vi "Overview.vi"() -> ()   [LabVIEW 2024]
uses:
  Overview_States.ctl
  State Data.ctl
  <vilib>/Plug-In SDKs/Clients/Metadata/Operator.ctl
  <vilib>/Plug-In SDKs/Clients/Metadata/Extension Value.ctl
  <vilib>/Plug-In SDKs/Clients/Metadata/Test Station.ctl
  <vilib>/Plug-In SDKs/Clients/Metadata/Software Item.ctl
  <vilib>/Plug-In SDKs/Clients/Data Store V1/Data Store Client.lvlibp/API/Data Store V1/Test Result.ctl
  <vilib>/Plug-In SDKs/Clients/Metadata/Outcome.ctl
  <vilib>/Plug-In SDKs/Clients/Metadata/Error Information.ctl
  <vilib>/Plug-In SDKs/Clients/Metadata/Step.ctl
  <vilib>/Plug-In SDKs/Clients/Metadata Store V1/Metadata Store Client.lvlibp/API/Metadata Store V1/Register Schema (Path).vi
  <vilib>/Plug-In SDKs/Clients/Metadata Store V1/Metadata Store Client.lvlibp/API/Metadata Store V1/Create Operator.vi
  <vilib>/Plug-In SDKs/Clients/Metadata Store V1/Metadata Store Client.lvlibp/API/Metadata Store V1/Create Alias (Metadata - Operator).vi
  <vilib>/Plug-In SDKs/Clients/Metadata Store V1/Metadata Store Client.lvlibp/API/Metadata Store V1/Create Test Station.vi
  <vilib>/Plug-In SDKs/Clients/Metadata Store V1/Metadata Store Client.lvlibp/API/Metadata Store V1/Create Software Item.vi
  <vilib>/Plug-In SDKs/Clients/Metadata Store V1/Metadata Store Client.lvlibp/API/Metadata Store V1/Query Test Stations.vi
  <vilib>/Plug-In SDKs/Clients/Data Store V1/Data Store Client.lvlibp/API/Data Store V1/Publish Measurement (DBL Analog Waveform).vi
  <vilib>/Plug-In SDKs/Clients/Metadata Store V1/Metadata Store Client.lvlibp/API/Metadata Store V1/Get Operator.vi
  <vilib>/Plug-In SDKs/Clients/Data Store V1/Data Store Client.lvlibp/API/Data Store V1/Read Data from Measurement (DBL Analog Waveform).vi
  <vilib>/Plug-In SDKs/Clients/Metadata Store V1/Metadata Store Client.lvlibp
  <vilib>/Plug-In SDKs/Clients/Data Store V1/Data Store Client.lvlibp
  <vilib>/Plug-In SDKs/Clients/Metadata/NI Metadata Types.lvlib
  <vilib>/measure/NI_MABase.lvlib
panel:
  out "queried data":waveform(dbl)(graph)
  out "log":string
  out "error out":errorcluster
  # "Overview\n\nThis example publishes a waveform along with metadata and extension attributes.\nThen it queries for the published data and displays it."
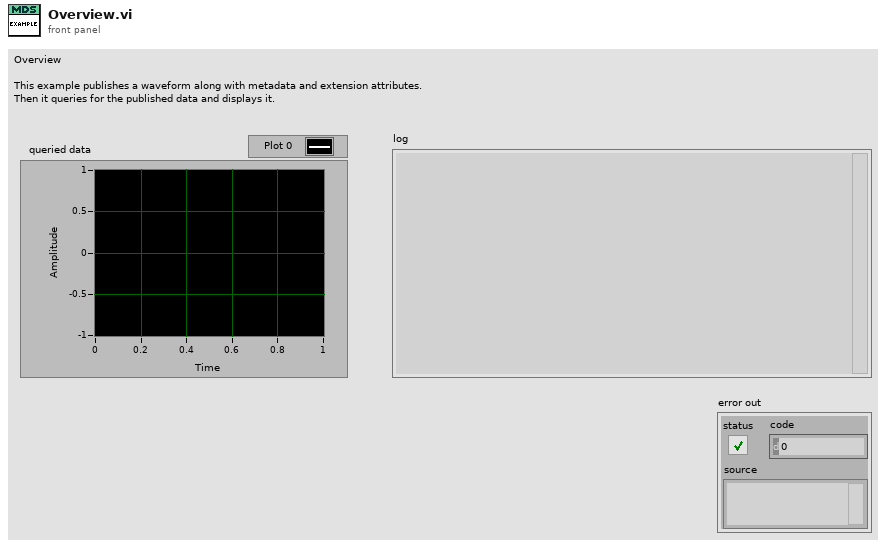
[diagram p1: front panel]
types:
  T1 = typedef "State Data.ctl" = cluster{"schema id":string, "software item ids":string[], "test result id":string, "published measurement id":string}
  T2 = typedef "Overview_States.ctl" = enum16{"Register Metadata Schema", "Create Metadata", "Create Test Result", "Publish Data", "Query Published Data"}
  T3 = enum16{"Register Metadata Schema", "Create Metadata", "Create Test Result", "Publish Data", "Query Published Data"}
  T4 = typedef "NI Metadata Types.lvlib/Extension Value.ctl" = cluster{"name":string, "value":string}
  T5 = typedef "NI Metadata Types.lvlib/Software Item.ctl" = cluster{"product":string, "version":string, "id":string, "link":string, "extension":T4[], "schema id":string}
  T6 = typedef "NI Metadata Types.lvlib/Test Station.ctl" = cluster{"name":string, "asset identifier":string, "id":string, "link":string, "extension":T4[], "schema id":string}
  T7 = typedef "NI Metadata Types.lvlib/Operator.ctl" = cluster{"name":string, "role":string, "id":string, "link":string, "extension":T4[], "schema id":string}
  T8 = typedef "Data Store Client.lvlibp/Test Result.ctl" = cluster{"name":string, "start date time":timestamp, "end date time":timestamp, "outcome":T9, "error information":T10, "id":string, "uut instance id":string, "operator id":string, "test station id":string, "test description id":string, "software item ids":string[], "hardware item ids":string[], "test adapter ids":string[], "link":string, "extension":T4[], "schema id":string}
  T9 = typedef "NI Metadata Types.lvlib/Outcome.ctl" = enum32{"Unspecified", "Passed", "Failed", "Indeterminate"}
  T10 = typedef "NI Metadata Types.lvlib/Error Information.ctl" = cluster{"error code":i32, "message":string, "source":string}
  T11 = typedef "NI Metadata Types.lvlib/Step.ctl" = cluster{"name":string, "step type":string, "start date time":timestamp, "end date time":timestamp, "notes":string, "outcome":T9, "error information":T10, "id":string, "parent step id":string, "test result id":string, "test id":string, "link":string, "extension":T4[], "schema id":string}
  T12 = typedef "Data Store Client.lvlibp/Published Measurement.ctl" = cluster{"parametric index":i32, "name":string, "value type":string, "notes":string, "start date time":timestamp, "end date time":timestamp, "outcome":T9, "error information":T10, "published conditions":T13[], "data moniker":T14, "id":string, "test result id":string, "step id":string, "software item ids":string[], "hardware item ids":string[], "test adapter ids":string[]}
  T13 = typedef "Data Store Client.lvlibp/Published Condition.ctl" = cluster{"name":string, "condition type":string, "moniker":T14, "id":string, "step id":string, "test result id":string}
  T14 = typedef "Data Store Client.lvlibp/Data Moniker.ctl" = cluster{"service location":string, "data source":string, "data instance":i64}
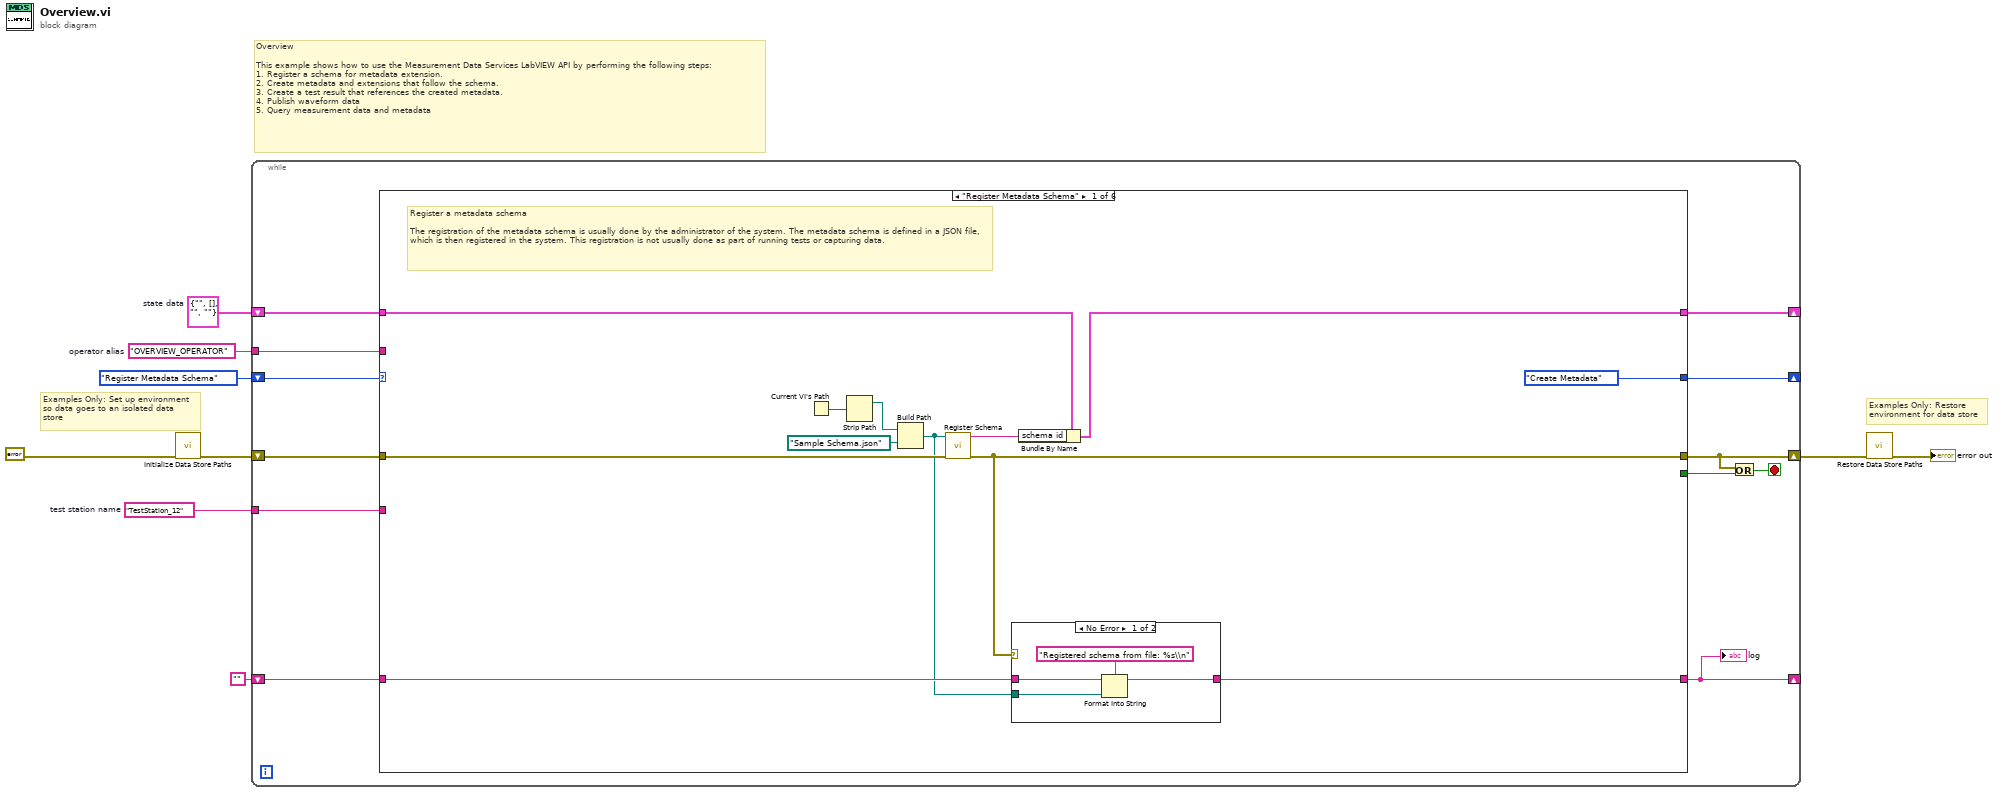
[diagram p0: block diagram]
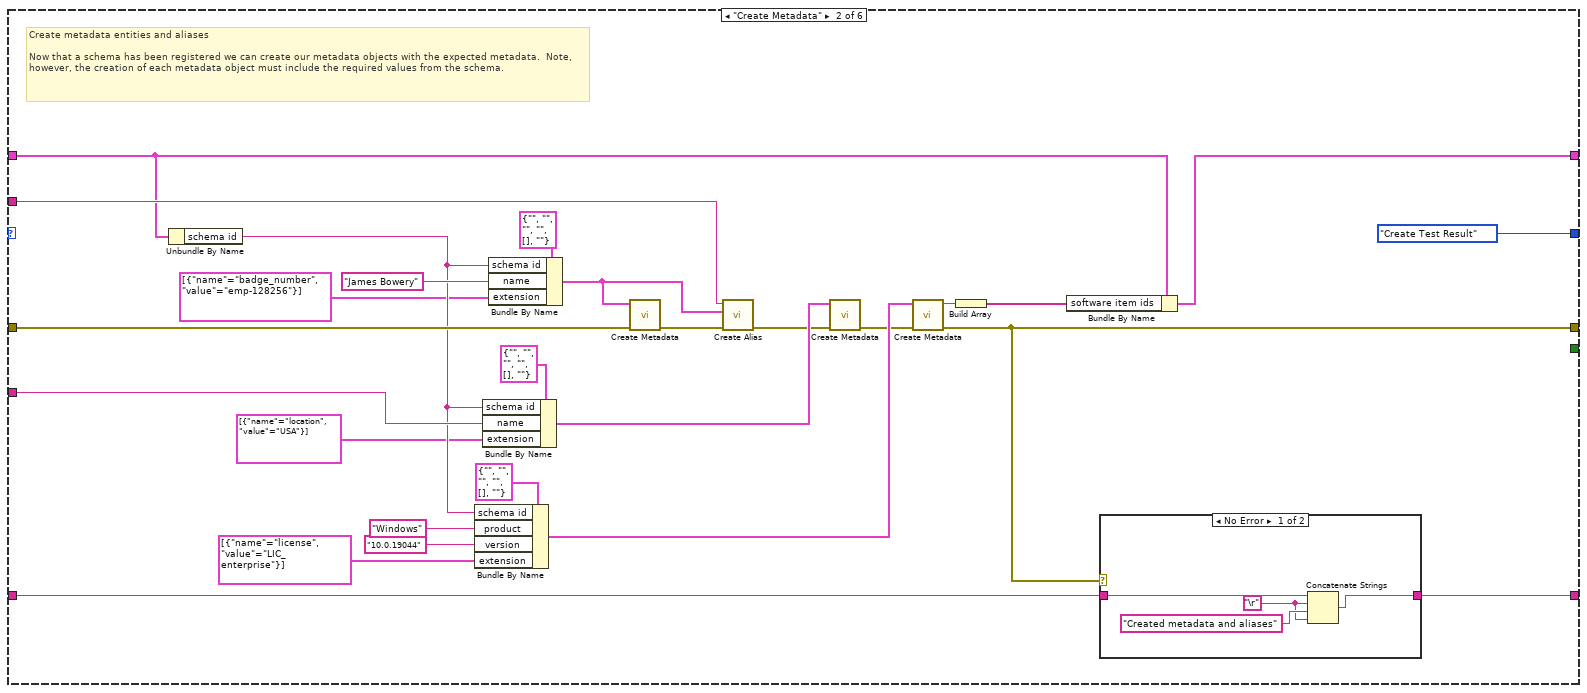
[diagram p3: hidden frame]
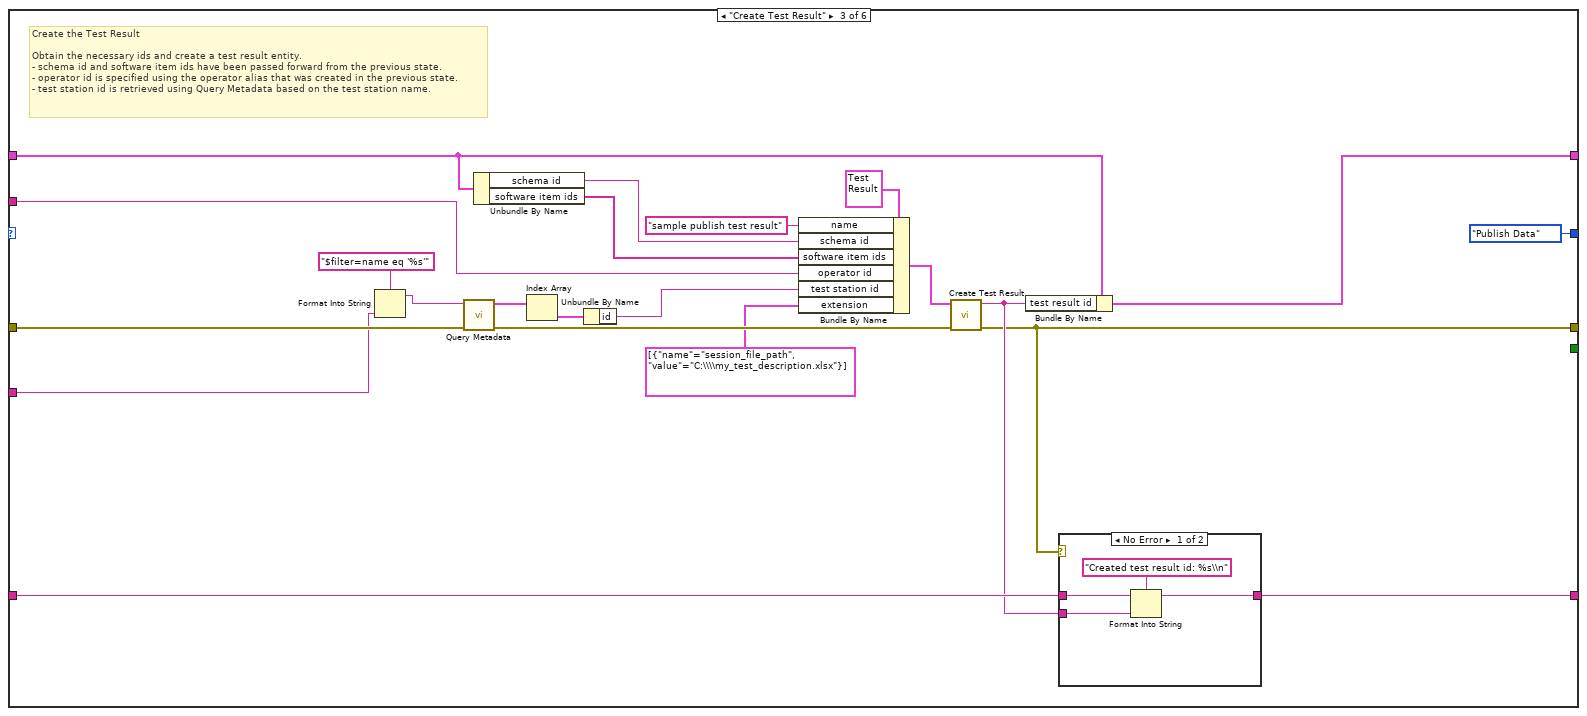
[diagram p5: hidden frame]
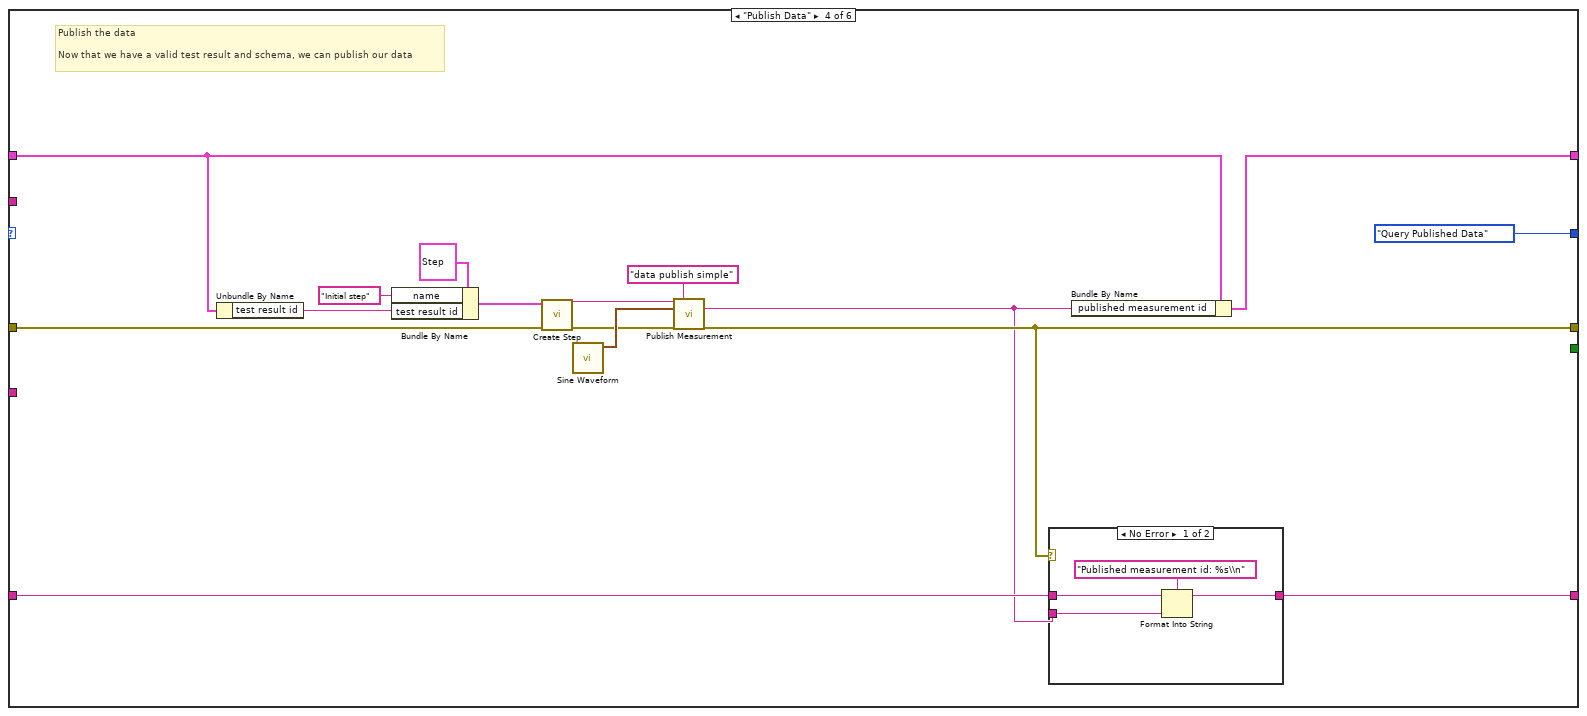
[diagram p7: hidden frame]
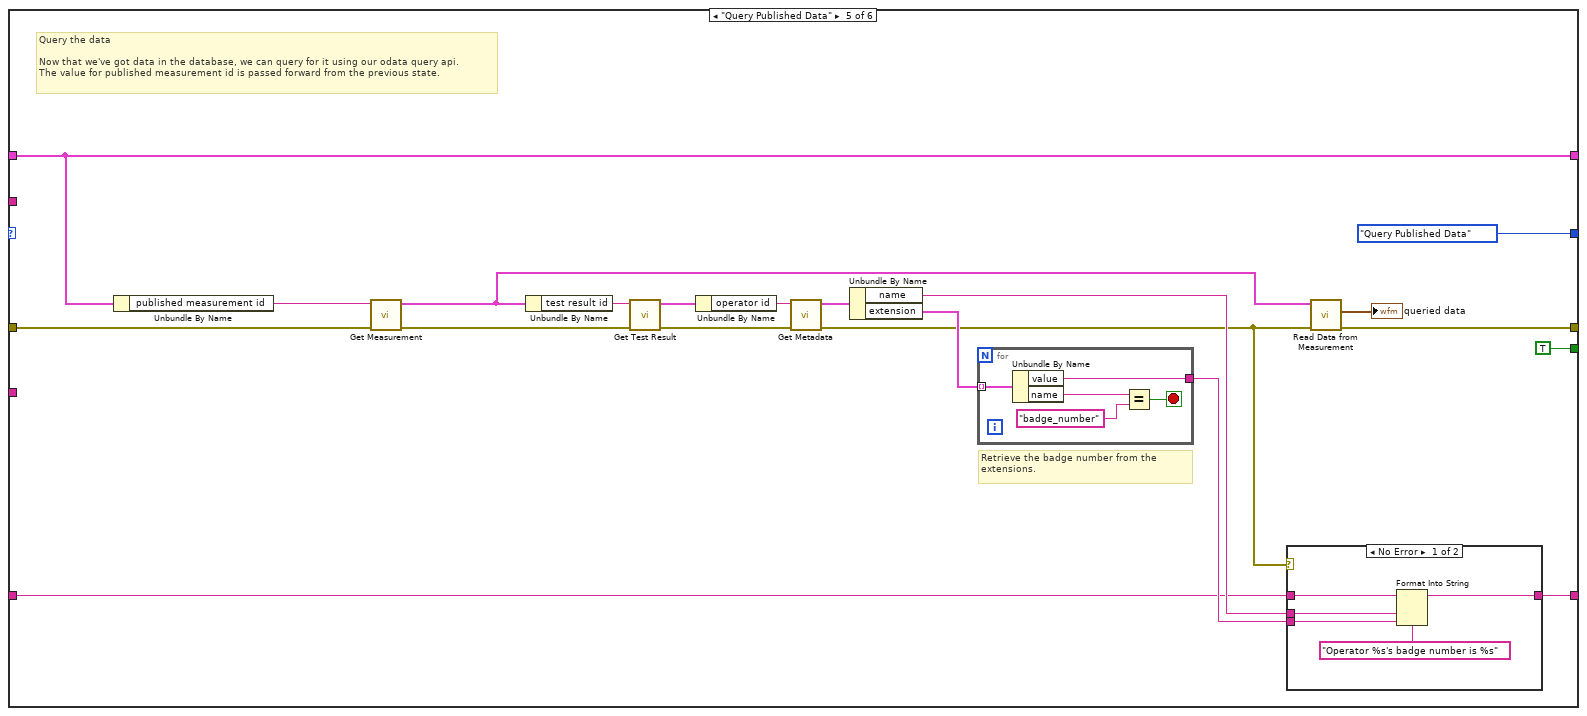
[diagram p9: hidden frame]
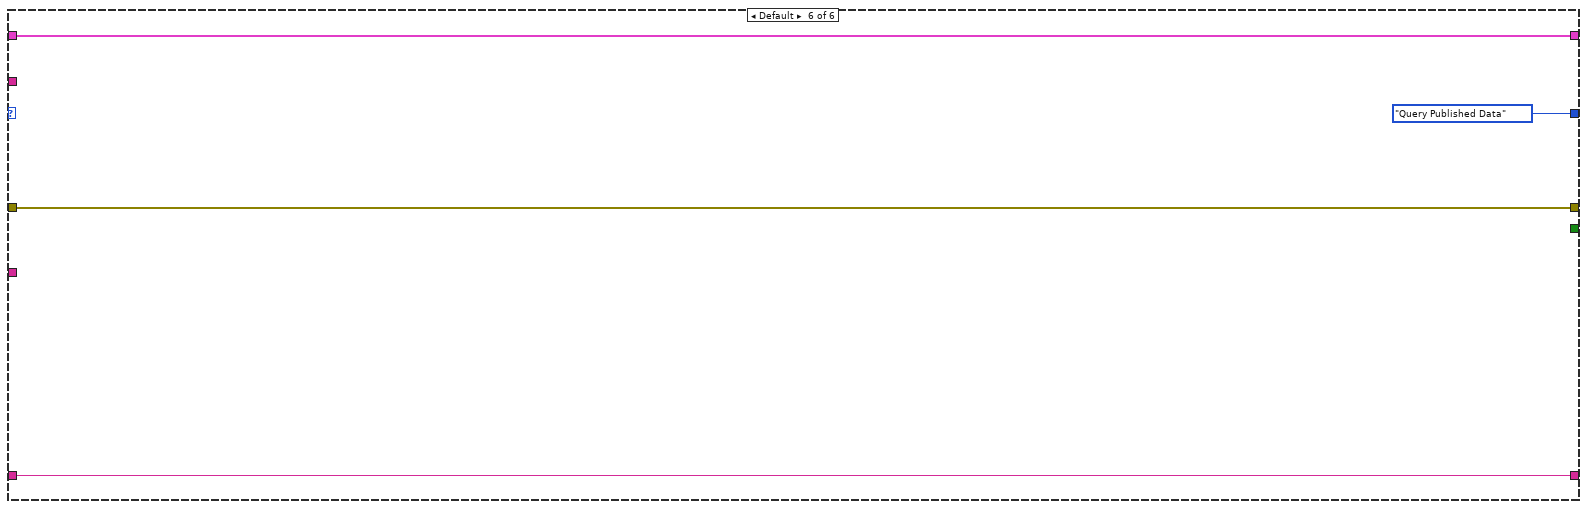
[diagram p11: hidden frame]
diagram:
  w5 = "OVERVIEW_OPERATOR"  # operator alias
  w6 = "TestStation_12"  # test station name
  w7 = T1 {"schema id"="", "software item ids"=[], "test result id"="", "published measurement id"=""}  # state data
  # "Examples Only: Restore\nenvironment for data store"
  # "Examples Only: Set up environment\nso data goes to an isolated data\nstore"
  # "Overview\n\nThis example shows how to use the Measurement Data Services LabVIEW API by performing the following steps:\n1. Register a schema for metadata extension.\n2. Create metadata and extensions that follow the schema.\n3. Create a test result that references the created metadata.\n4. Publish waveform data\n5. Query measurement data and metadata"
  n1 = call "Initialize Data Store Paths.vi"("error in"=errorcluster {"status"=FALSE, "code"=0, "source"=""} ("error out")) -> ("error out"=w3:errorcluster)  [unwired: 10 in]
  n2 = while {
    shift-right: [w18] -> _
    shift-left: Overview_States."Register Metadata Schema" ("state variable") -> [w21]
    shift-right: [w16] -> w2
    shift-left: w3 -> [w20]
    shift-right: [w17] -> _
    shift-left: "" ("log") -> [w19]
    shift-right: [w10] -> _
    shift-left: w7 -> [w13]
    tunnel: w6 -> [w12]
    tunnel: w5 -> [w11]
    stop <- w14 stop-if-true
    n3 = case shown="\"Register Metadata Schema\"" w21 {
      tunnel: [w27 w44 w75 w103 w138 w153] -> w16
      tunnel: w20 -> [w28 w65 w85 w106 w121 w153]
      tunnel: [w29 w42 w90 w107 w126 w152] -> w17
      tunnel: w19 -> [w30 w43 w89 w104 w127 w152]
      tunnel: [T3."Create Metadata" T3."Create Test Result" T3."Publish Data" T3."Query Published Data" T3."Query Published Data" T3."Query Published Data"] -> w18
      tunnel: [_ _ _ _ TRUE _] -> w15
      tunnel: w13 -> [w24 w47 w78 w100 w123 w150]
      tunnel: w12 -> [_ w53 w81 _ _ _]
      tunnel: w11 -> [_ w49 w73 _ _ _]
      tunnel: [w22 w45 w87 w101 w123 w150] -> w10
      frame "Register Metadata Schema" {
        # "Register a metadata schema\n\nThe registration of the metadata schema is usually done by the administrator of the system. The metadata schema is defined in a JSON file, which is then registered in the system. This registration is not usually done as part of running tests or capturing data."
        n4 = Current VI's Path() -> (path=w33:path)
        n5 = Strip Path(path=w33) -> (stripped path=w32:path)  [unwired: 1 out]
        n6 = Build Path(base path=w32, name or relative path=path "Sample Schema.json") -> (appended path=w26:path)
        n7 = call-poly <vilib>:"Register Schema.vi"("error in"=w28, "schema"=w26) -> ("error out"=w27:errorcluster, "schema id"=w23:string)  [unwired: 8 in]
        n8 = case shown="No Error" w27 {
          tunnel: w30 -> [w37 w38]
          tunnel: [w36 w38] -> w29
          tunnel: w26 -> [w35 _]
          frame No Error {
            n9 = Format Into String(format string="Registered schema from file: %s\\n", initial string=w37, w35) -> (resulting string=w36:string)  [unwired: 1 in, 1 out]
          }
          frame Error {
          }
        }
        n10 = Bundle By Name(cluster=w24, "schema id"=w23) -> (w22:T1)
      }
      frame "Create Metadata" {
        # "Create metadata entities and aliases\n\nNow that a schema has been registered we can create our metadata objects with the expected metadata.  Note, however, the creation of each metadata object must include the required values from the schema."
        n11 = Unbundle By Name(w47) -> ("schema id"=w50:string)
        n12 = Bundle By Name(cluster=T5 {"product"="", "version"="", "id"="", "link"="", "extension"=[], "schema id"=""} ("software item"), "schema id"=w50, "product"="Windows", "version"="10.0.19044", "extension"=T4[] [{"name"="license", "value"="LIC_enterprise"}]) -> (w58:T5)
        n13 = Bundle By Name(cluster=T6 {"name"="", "asset identifier"="", "id"="", "link"="", "extension"=[], "schema id"=""} ("test station"), "schema id"=w50, "name"=w53, "extension"=T4[] [{"name"="location", "value"="USA"}]) -> (w56:T6)
        n14 = Bundle By Name(cluster=T7 {"name"="", "role"="", "id"="", "link"="", "extension"=[], "schema id"=""} ("operator metadata"), "schema id"=w50, "name"="James Bowery" ("operator name"), "extension"=T4[] [{"name"="badge_number", "value"="emp-128256"}]) -> (w51:T7)
        n15 = call-poly <vilib>:"Create Metadata.vi"("error in"=w65, "operator metadata"=w51) -> ("error out"=w52:errorcluster)  [unwired: 8 in, 1 out]
        n16 = call-poly <vilib>:"Create Alias.vi"("error in"=w52, "operator"=w51, "alias name"=w49) -> ("error out"=w48:errorcluster)  [unwired: 7 in, 1 out]
        n17 = call-poly <vilib>:"Create Metadata.vi"("error in"=w48, "test station"=w56) -> ("error out"=w57:errorcluster)  [unwired: 8 in, 1 out]
        n18 = call-poly <vilib>:"Create Metadata.vi"("error in"=w57, "software item"=w58) -> ("error out"=w44:errorcluster, "software item id"=w64:string)  [unwired: 8 in]
        n19 = Build Array(w64) -> (w46:string[])
        n20 = Bundle By Name(cluster=w47, "software item ids"=w46) -> (w45:T1)
        n21 = case shown="No Error" w44 {
          tunnel: w43 -> [w69 w70]
          tunnel: [w66 w70] -> w42
          frame No Error {
            w67 = "\r"
            n22 = Concatenate Strings(w69, w67, "Created metadata and aliases" ("string"), w67) -> (w66:string)
          }
          frame Error {
          }
        }
      }
      frame "Create Test Result" {
        # "Create the Test Result\n\nObtain the necessary ids and create a test result entity.\n- schema id and software item ids have been passed forward from the previous state.\n- operator id is specified using the operator alias that was created in the previous state.\n- test station id is retrieved using Query Metadata based on the test station name."
        n23 = Format Into String(format string="$filter=name eq '%s'", w81) -> (resulting string=w79:string)  [unwired: 2 in, 1 out]
        n24 = call-poly <vilib>:"Query Metadata.vi"("error in"=w85, "odata query"=w79) -> ("error out"=w84:errorcluster, "test stations"=w83:T6[])  [unwired: 8 in]
        n25 = Unbundle By Name(w78) -> ("schema id"=w77:string, "software item ids"=w72:string[])
        n26 = Index Array(array=w83) -> (element=w82:T6)  [unwired: 1 in]
        n27 = Unbundle By Name(w82) -> ("id"=w76:string)
        n28 = Bundle By Name(cluster=T8 {"name"="", "start date time"=timestamp(0 s since 1904-01-01), "end date time"=timestamp(0 s since 1904-01-01), "outcome"=enum."Unspecified", "error information"={"error code"=0, "message"="", "source"=""}, "id"="", "uut instance id"="", "operator id"="", "test station id"="", "test description id"="", "software item ids"=[], "hardware item ids"=[], "test adapter ids"=[], "link"="", "extension"=[], "schema id"=""} ("test result"), "name"="sample publish test result" ("test result name"), "schema id"=w77, "software item ids"=w72, "operator id"=w73, "test station id"=w76, "extension"=T4[] [{"name"="session_file_path", "value"="C:\\\\my_test_description.xlsx"}]) -> (w92:T8)
        n29 = call <vilib>:"Create Test Result.vi"("error in"=w84, "test result"=w92) -> ("error out"=w75:errorcluster, "test result id"=w86:string)  [unwired: 8 in]
        n30 = Bundle By Name(cluster=w78, "test result id"=w86) -> (w87:T1)
        n31 = case shown="No Error" w75 {
          tunnel: w89 -> [w95 w97]
          tunnel: [w94 w97] -> w90
          tunnel: w86 -> [w93 _]
          frame No Error {
            n32 = Format Into String(format string="Created test result id: %s\\n", initial string=w95, w93) -> (resulting string=w94:string)  [unwired: 1 in, 1 out]
          }
          frame Error {
          }
        }
      }
      frame "Publish Data" {
        # "Publish the data\n\nNow that we have a valid test result and schema, we can publish our data"
        n33 = Unbundle By Name(w100) -> ("test result id"=w99:string)
        n34 = Bundle By Name(cluster=T11 {"name"="", "step type"="", "start date time"=timestamp(0 s since 1904-01-01), "end date time"=timestamp(0 s since 1904-01-01), "notes"="", "outcome"=enum."Unspecified", "error information"={"error code"=0, "message"="", "source"=""}, "id"="", "parent step id"="", "test result id"="", "test id"="", "link"="", "extension"=[], "schema id"=""} ("step"), "name"="Initial step" ("step name"), "test result id"=w99) -> (w111:T11)
        n35 = call <vilib>:"Create Step.vi"("error in"=w106, "step"=w111) -> ("error out"=w110:errorcluster, "step id"=w109:string)  [unwired: 8 in]
        n36 = call <vilib>:"Sine Waveform.vi"() -> ("signal out"=w113:waveform(dbl))  [unwired: 10 in, 1 out]
        n37 = call-poly <vilib>:"Publish Measurement.vi"("step id"=w109, "name"="data publish simple", "waveform"=w113, "error in"=w110) -> ("measurement id"=w98:string, "error out"=w103:errorcluster)  [unwired: 9 in, 1 out]
        n38 = case shown="No Error" w103 {
          tunnel: w98 -> [w117 _]
          tunnel: [w115 w118] -> w107
          tunnel: w104 -> [w114 w118]
          frame No Error {
            n39 = Format Into String(format string="Published measurement id: %s\\n", initial string=w114, w117) -> (resulting string=w115:string)  [unwired: 1 in, 1 out]
          }
          frame Error {
          }
        }
        n40 = Bundle By Name(cluster=w100, "published measurement id"=w98) -> (w101:T1)
      }
      frame "Query Published Data" {
        # "Query the data\n\nNow that we've got data in the database, we can query for it using our odata query api.\nThe value for published measurement id is passed forward from the previous state."
        # "Retrieve the badge number from the extensions."
        n41 = Unbundle By Name(w123) -> ("published measurement id"=w122:string)
        n42 = call <vilib>:"Get Measurement.vi"("error in"=w121, "measurement id"=w122) -> ("error out"=w119:errorcluster, "published measurement"=w120:T12)  [unwired: 8 in]
        n43 = Unbundle By Name(w120) -> ("test result id"=w132:string)
        n44 = call <vilib>:"Get Test Result.vi"("error in"=w119, "test result id"=w132) -> ("error out"=w131:errorcluster, "test result"=w130:T8)  [unwired: 8 in]
        n45 = Unbundle By Name(w130) -> ("operator id"=w129:string)
        n46 = call-poly <vilib>:"Get Metadata.vi"("error in"=w131, "operator id"=w129) -> ("error out"=w125:errorcluster, "operator metadata"=w128:T7)  [unwired: 8 in]
        n47 = Unbundle By Name(w128) -> ("name"=w133:string, "extension"=w134:T4[])
        n48 = for {
          tunnel: w134 -> [w149] mode=indexing
          tunnel: [w145] -> w135
          stop <- w146 stop-if-true
          n49 = Unbundle By Name(w149) -> ("value"=w145:string, "name"=w148:string)
          n50 = Equal?(x=w148, y="badge_number") -> (x = y?=w146:bool)
        }
        n51 = case shown="No Error" w125 {
          tunnel: w135 -> [w143 _]
          tunnel: w133 -> [w142 _]
          tunnel: w127 -> [w140 w144]
          tunnel: [w139 w144] -> w126
          frame No Error {
            n52 = Format Into String(format string="Operator %s's badge number is %s", initial string=w140, w142, w143) -> (resulting string=w139:string)  [unwired: 1 in, 1 out]
          }
          frame Error {
          }
        }
        n53 = call-poly <vilib>:"Read Data from Measurement.vi"("error in"=w125, "published measurement"=w120) -> ("error out"=w138:errorcluster, "waveform data"=→"queried data":waveform(dbl))  [unwired: 7 in, 1 out]
      }
      frame Default {
      }
    }
    "log" <- w17
    n54 = Or(x=w16, y=w15) -> (x .or. y?=w14:bool)
  }
  n55 = call "Restore Data Store Paths.vi"("error in"=w2) -> ("error out"=→"error out":errorcluster)  [unwired: 10 in]
